vi "poly.vi"   [LabVIEW 2020]
uses:
  common/file Viewer/FV-file_viewer.lvlib
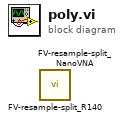
[diagram p0: block diagram]
diagram:
  n1 = call "FV-resample-split_R140.vi"() -> ()  [unwired: 10 in, 2 out]
  n2 = call "FV-resample-split_NanoVNA.vi"() -> ()  [unwired: 11 in, 1 out]
